vi "SetPosition.vi"(8 "error in (no error)":errorcluster, 9 "coordinates":dbl[](array[numeric]), 10 "name":string, 11 "DirectedGraphMapNode in":refnum<class "NI_Robotics_DirectedGraphMapNode.lvclass">) -> (0 "error out":errorcluster, 3 "DirectedGraphMapNode out":refnum<class "NI_Robotics_DirectedGraphMapNode.lvclass">)   [LabVIEW 2017, in "NI_Robotics_DirectedGraphMapNode.lvclass"]
uses:
  <vilib>/robotics/Navigation/shared/MapNode/DirectedGraphMapNode/NI_Robotics_DirectedGraphMapNode.lvclass
  <vilib>/robotics/Navigation/shared/MapNode/DirectedGraphMapNode/NI_Robotics_DirectedGraphMapNode.lvclass/NI_Robotics_DirectedGraphMapNode.ctl
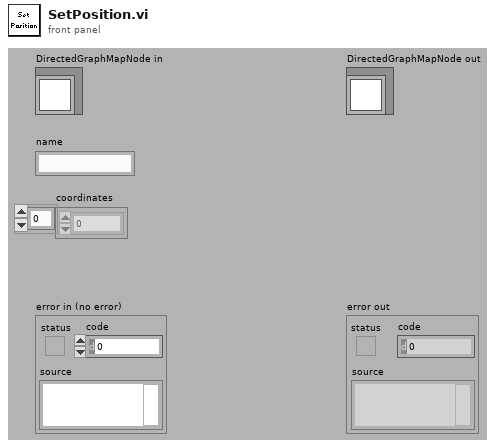
[diagram p1: front panel]
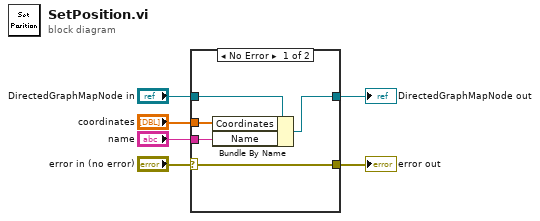
[diagram p0: block diagram]
diagram:
  n1 = case shown="No Error" "error in (no error)" {
    selector: "error in (no error)" -> [w11 w13]
    tunnel: [w11 w13] -> w5
    tunnel: [w9 w12] -> w3
    tunnel: "DirectedGraphMapNode in" -> [w10 w12]
    tunnel: "coordinates" -> [w8 _]
    tunnel: "name" -> [w7 _]
    frame No Error {
      n2 = Bundle By Name(cluster=w10, "Coordinates"=w8, "Name"=w7) -> (w9:refnum<class "NI_Robotics_DirectedGraphMapNode.lvclass">)
    }
    frame Error {
    }
  }
  "error out" <- w5
  "DirectedGraphMapNode out" <- w3
